vi "Export Waveforms To Spreadsheet File with modified timestamps.vi"(0 "file path (dialog if empty)":path, 1 "prompt":string="Choose file to write.", 3 "delimiter (Tab)":string="\t", 5 "waveforms":waveform(dbl)[](array[waveform]), 7 "error in (no error)":errorcluster, 9 "multiple time columns? (single:F)":bool, 11 "trial start time":timestamp, 12 "append to file? (new file:F)":bool, 14 "header? (write header:T)":bool=TRUE) -> (4 "new file path (Not A Path if cancelled)":path, 15 "error out":errorcluster)   [LabVIEW 2016]
doc: "Converts a waveform to a text string and writes the string to a new byte stream file or appends the string to an existing file. Wire data to the <B>waveforms</B> input to determine the polymorphic instance to use or manually select the instance."
uses:
  <vilib>/Waveform/WDTOps.llb/WDT Get Waveform Time Array DBL.vi
panel:
  out "Array":string[](array[string])
  out "spreadsheet string":string
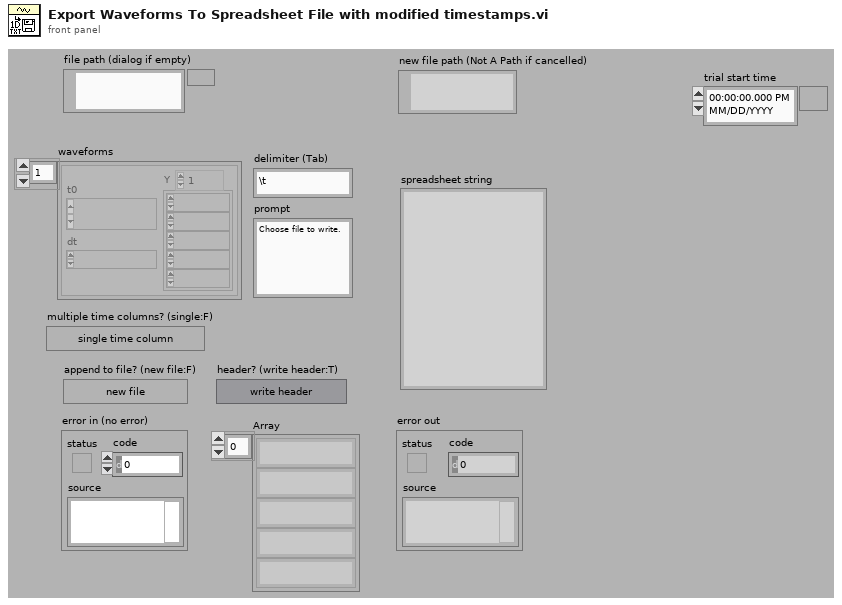
[diagram p1: front panel]
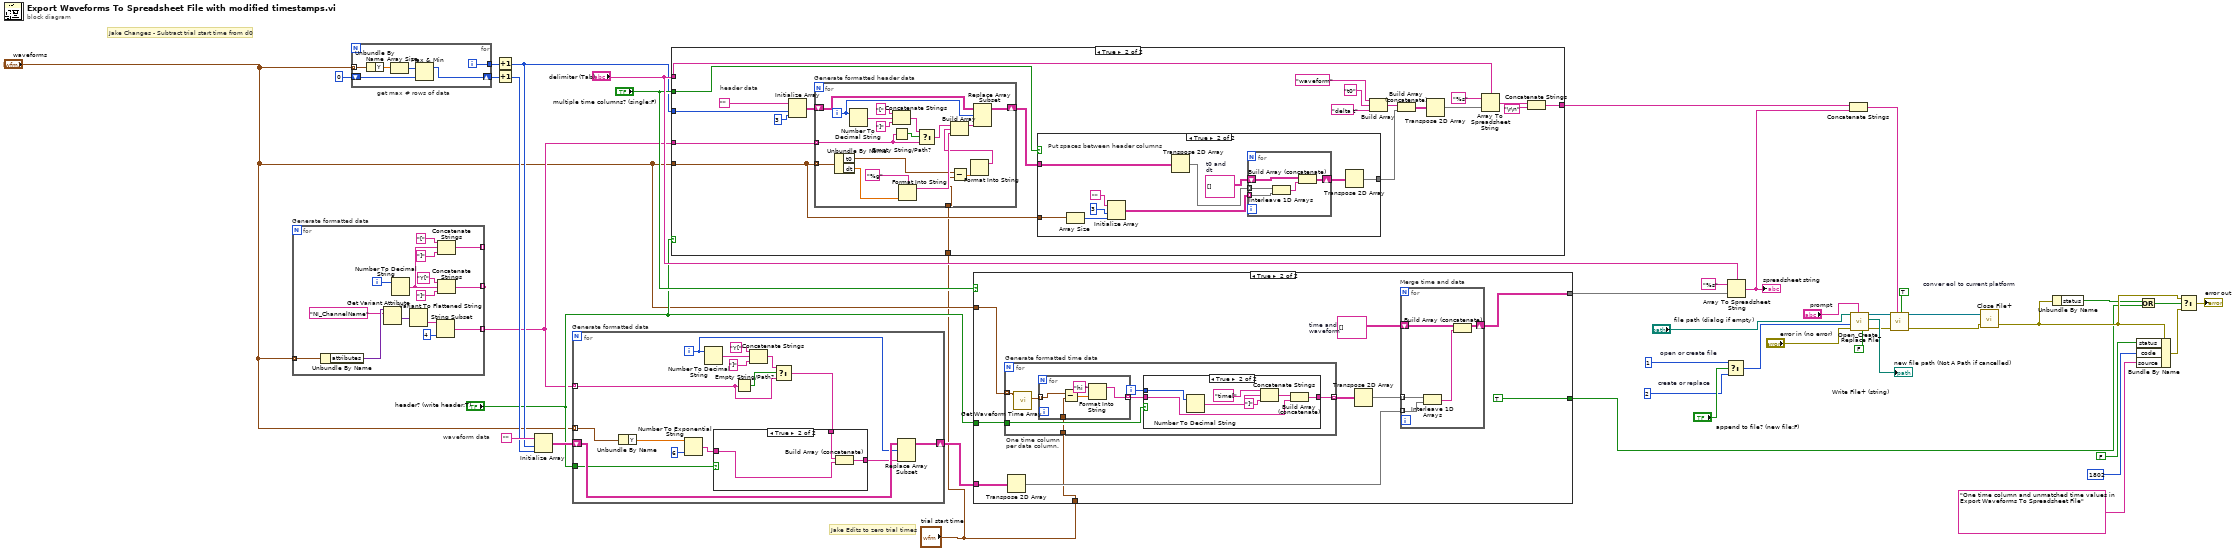
[diagram p0: block diagram]
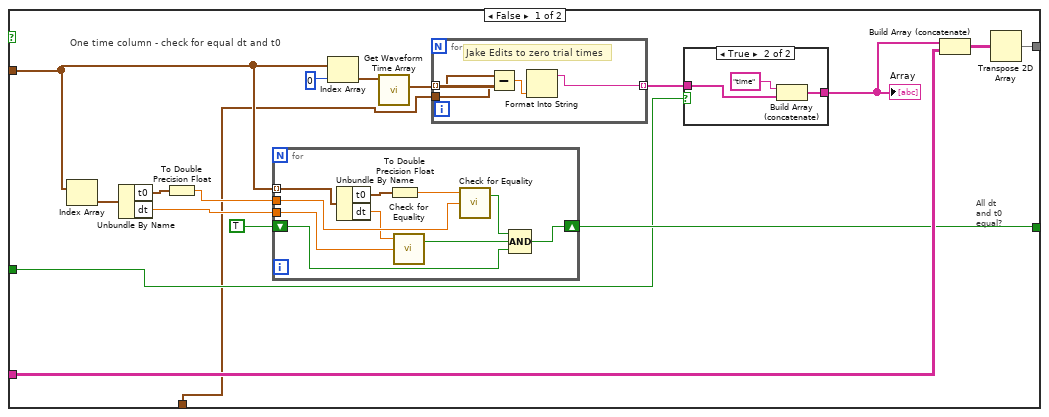
[diagram p2: hidden frame]
diagram:
  w34 = i16 2  # create or replace
  w36 = TRUE  # conver eol to current platform
  w41 = i16 1  # open or create file
  # "Jake Edits to zero trial times"
  # "Jake Changes - Subtract trial start time from d0"
  # "waveform data"
  # "get max # rows of data"
  n1 = for "Generate formatted data" {
    tunnel: "waveforms" -> [w57] mode=indexing
    tunnel: [w48] -> _ mode=indexing
    tunnel: [w47] -> w5 mode=indexing
    tunnel: [w43] -> _ mode=indexing
    i -> [w49]
    n2 = Unbundle By Name(w57) -> ("attributes"=w54:variant)
    n3 = Get Variant Attribute(Variant=w54, name="NI_ChannelName") -> (value=w52:variant)  [unwired: 2 in, 3 out]
    n4 = Number To Decimal String(number=w49) -> (decimal integer string=w44:string)  [unwired: 1 in]
    n5 = Variant To Flattened String(Variant=w52) -> (data string=w55:string)  [unwired: 1 out]
    n6 = String Subset(string=w55, offset (0)=4) -> (substring=w47:string)  [unwired: 1 in]
    n7 = Concatenate Strings("[", w44, "]") -> (w43:string)
    n8 = Concatenate Strings("Y[", w44, "]") -> (w48:string)
  }
  n9 = for {
    tunnel: "waveforms" -> [w63] mode=indexing
    shift-right: [w59] -> w11
    shift-left: 0 -> [w60]
    tunnel: [w58] -> w9
    i -> [w58]
    n10 = Unbundle By Name(w63) -> ("Y"=w62:dbl[])
    n11 = Array Size(array=w62) -> (size(s)=w61:i32)
    n12 = Max & Min(x=w61, y=w60) -> (max(x,y)=w59:i32)  [unwired: 1 out]
  }
  n13 = Increment(x=w9) -> (x+1=w8:i32)
  n14 = Increment(x=w11) -> (x+1=w7:i32)
  n15 = Initialize Array("", w8, w7) -> (w10:string[][])
  n16 = for "Generate formatted data" {
    tunnel: "waveforms" -> [w77] mode=indexing
    tunnel: "header? (write header:T)" -> [w74]
    shift-right: [w75] -> w25
    shift-left: w10 -> [w76]
    tunnel: w5 -> [w64] mode=indexing
    i -> [w66]
    n17 = Unbundle By Name(w77) -> ("Y"=w79:dbl[])
    n18 = Number To Exponential String(number=w79, precision (6)=i16 6) -> (E-format string=w73:string[])  [unwired: 2 in]
    n19 = Number To Decimal String(number=w66) -> (decimal integer string=w71:string)  [unwired: 1 in]
    n20 = Empty String/Path?(string/path=w64) -> (empty?=w68:bool)
    n21 = Concatenate Strings("Y[", w71, "]") -> (w65:string)
    n22 = Select(t=w65, s=w68, f=w64) -> (s? t:f=w67:string)
    n23 = case shown="True" w74 {
      tunnel: w73 -> [w80 w83]
      tunnel: [w80 w82] -> w72
      tunnel: w67 -> [_ w81]
      frame False {
      }
      frame True {
        n24 = Build Array (concatenate)(w81, w83) -> (w82:string[])
      }
    }
    n25 = Replace Array Subset(array=w76, new element=w72, index (row)=w66) -> (w75:string[][])  [unwired: 1 in]
  }
  n26 = case shown="True" "header? (write header:T)" {
    tunnel: "delimiter (Tab)" -> [_ w102]
    tunnel: "waveforms" -> [_ w96]
    tunnel: [_ w97] -> w26
    tunnel: "multiple time columns? (single:F)" -> [_ w94]
    tunnel: w8 -> [_ w87]
    tunnel: w5 -> [_ w85]
    tunnel: "trial start time" -> [_ w84]
    frame False {
    }
    frame True {
      # "header data"
      n27 = Initialize Array("", w87, 3 ("dimension size")) -> (w86:string[][])
      n28 = for "Generate formatted header data" {
        tunnel: w96 -> [w134] mode=indexing
        shift-right: [w130] -> w92
        shift-left: w86 -> [w131]
        tunnel: w85 -> [w125] mode=indexing
        tunnel: w84 -> [w123]
        i -> [w129]
        n29 = Unbundle By Name(w134) -> ("t0"=w122:timestamp, "dt"=w138:dbl)
        n30 = Number To Decimal String(number=w129) -> (decimal integer string=w137:string)  [unwired: 1 in]
        n31 = Concatenate Strings("[", w137, "]") -> (w128:string)
        n32 = Empty String/Path?(string/path=w125) -> (empty?=w126:bool)
        n33 = Format Into String(format string="%g" ("Format String"), w138) -> (resulting string=w139:string)  [unwired: 2 in, 1 out]
        n34 = Select(t=w128, s=w126, f=w125) -> (s? t:f=w127:string)
        n35 = Subtract(x=w122, y=w123) -> (x-y=w124:dbl)
        n36 = Format Into String(w124) -> (resulting string=w121:string)  [unwired: 3 in, 1 out]
        n37 = Build Array(w127, w121, w139) -> (w132:string[])
        n38 = Replace Array Subset(array=w131, new element=w132, index (row)=w129) -> (w130:string[][])  [unwired: 1 in]
      }
      n39 = case shown="True" w94 {
        tunnel: w96 -> [_ w115]
        tunnel: [w105 w110] -> w93
        tunnel: w92 -> [w105 w109]
        frame False {
          # "Leave the header data alone"
        }
        frame True {
          w113 = string[][] []  # t0 and dt
          # "Put spaces between header columns"
          n40 = Array Size(array=w115) -> (size(s)=w106:i32)
          n41 = Initialize Array("", 3 ("Dimension Size"), w106) -> (w112:string[][])
          n42 = Transpose 2D Array(2D array=w109) -> (transposed array=w108:string[][])
          n43 = for {
            shift-right: [w117] -> w111
            shift-left: w113 -> [w118]
            tunnel: w112 -> [w120] mode=indexing
            tunnel: w108 -> [w116] mode=indexing
            n44 = Interleave 1D Arrays(w116, w120) -> (w119:string[])
            n45 = Build Array (concatenate)(w118, w119) -> (w117:string[][])
          }
          n46 = Transpose 2D Array(2D array=w111) -> (transposed array=w110:string[][])
        }
      }
      n47 = Build Array("waveform", "t0", "delta t") -> (w95:string[])
      n48 = Build Array (concatenate)(w95, w93) -> (w90:string[][])
      n49 = Transpose 2D Array(2D array=w90) -> (transposed array=w91:string[][])
      n50 = Array To Spreadsheet String(delimiter (Tab)=w102, array=w91, 3:"%s" ("format string")) -> (spreadsheet string=w99:string)
      n51 = Concatenate Strings(w99, "\r\n") -> (w97:string)
    }
  }
  n52 = case shown="True" "multiple time columns? (single:F)" {
    tunnel: "waveforms" -> [w145 w184]
    tunnel: w25 -> [w152 w182]
    tunnel: [w150 w178] -> w24
    tunnel: [w144 TRUE] -> w14
    tunnel: "header? (write header:T)" -> [w141 w176]
    tunnel: "trial start time" -> [w140 w175]
    frame False {
      # "One time column - check for equal dt and t0"
      # "All dt\nand t0\nequal?"
      n53 = Index Array(array=w145) -> (element=w149:waveform(dbl))  [unwired: 1 in]
      n54 = Unbundle By Name(w149) -> ("t0"=w143:timestamp, "dt"=w146:dbl)
      n55 = To Double Precision Float(number=w143) -> (double precision float=w147:dbl)
      n56 = for {
        tunnel: w145 -> [w170] mode=indexing
        shift-right: [w165] -> w144
        shift-left: TRUE -> [w164]
        tunnel: w147 -> [w168]
        tunnel: w146 -> [w166]
        n57 = Unbundle By Name(w170) -> ("t0"=w161:timestamp, "dt"=w167:dbl)
        n58 = To Double Precision Float(number=w161) -> (double precision float=w169:dbl)
        n59 = call <vilib>:"Check for Equality.vi"("n2"=w166, "n1"=w167) -> ("equal?"=w163:bool)  [unwired: 1 in, 1 out]
        n60 = call <vilib>:"Check for Equality.vi"("n2"=w168, "n1"=w169) -> ("equal?"=w162:bool)  [unwired: 1 in, 1 out]
        n61 = Compound Arithmetic op=AND(w162, w163, w164) -> (w165:bool)
      }
      n62 = Index Array(array=w145, index=0 ("Index")) -> (element=w154:waveform(dbl))
      n63 = call-poly <vilib>:"Get Waveform Time Array.vi"("waveform in"=w154) -> ("X array"=w156:timestamp[])  [unwired: 9 in, 1 out]
      n64 = for {
        tunnel: w156 -> [w173] mode=indexing
        tunnel: [w171] -> w153 mode=indexing
        tunnel: w140 -> [w174]
        # "Jake Edits to zero trial times"
        n65 = Subtract(x=w173, y=w174) -> (x-y=w172:dbl)
        n66 = Format Into String(w172) -> (resulting string=w171:string)  [unwired: 3 in, 1 out]
      }
      n67 = case shown="True" w141 {
        tunnel: w153 -> [w157 w160]
        tunnel: [w157 w159] -> w142
        frame False {
        }
        frame True {
          n68 = Build Array (concatenate)("time", w160) -> (w159:string[])
        }
      }
      "Array" <- w142
      n69 = Build Array (concatenate)(w142, w152) -> (w151:string[][])
      n70 = Transpose 2D Array(2D array=w151) -> (transposed array=w150:string[][])
    }
    frame True {
      w179 = string[][] []  # time and waveform
      # "One time column\nper data column."
      n71 = for "Generate formatted time data" {
        tunnel: [w191] -> w183 mode=indexing
        tunnel: w184 -> [w195] mode=indexing
        tunnel: w176 -> [w193]
        tunnel: w175 -> [w190]
        i -> [w194]
        n72 = call-poly <vilib>:"Get Waveform Time Array.vi"("waveform in"=w195) -> ("X array"=w196:timestamp[])  [unwired: 9 in, 1 out]
        n73 = for {
          tunnel: w196 -> [w208] mode=indexing
          tunnel: [w206] -> w192 mode=indexing
          tunnel: w190 -> [w209]
          n74 = Subtract(x=w208, y=w209) -> (x-y=w207:dbl)
          n75 = Format Into String(initial string="hi ", w207) -> (resulting string=w206:string)  [unwired: 2 in, 1 out]
        }
        n76 = case shown="True" w193 {
          tunnel: w194 -> [_ w201]
          tunnel: w192 -> [w197 w199]
          tunnel: [w197 w198] -> w191
          frame False {
          }
          frame True {
            n77 = Number To Decimal String(number=w201) -> (decimal integer string=w204:string)  [unwired: 1 in]
            n78 = Concatenate Strings("time[", w204, "]") -> (w200:string)
            n79 = Build Array (concatenate)(w200, w199) -> (w198:string[])
          }
        }
      }
      n80 = Transpose 2D Array(2D array=w182) -> (transposed array=w181:string[][])
      n81 = Transpose 2D Array(2D array=w183) -> (transposed array=w180:string[][])
      n82 = for "Merge time and data" {
        tunnel: w181 -> [w188] mode=indexing
        tunnel: w180 -> [w187] mode=indexing
        shift-right: [w186] -> w178
        shift-left: w179 -> [w189]
        n83 = Interleave 1D Arrays(w187, w188) -> (w185:string[])
        n84 = Build Array (concatenate)(w189, w185) -> (w186:string[][])
      }
    }
  }
  n85 = Select ("function")(t=w41, s="append to file? (new file:F)", f=w34) -> (s? t:f=w39:i16)
  n86 = Array To Spreadsheet String(delimiter (Tab)="delimiter (Tab)", array=w24, 3:"%s" ("format (%.3f)")) -> (spreadsheet string=w27:string)
  "spreadsheet string" <- w27
  n87 = Concatenate Strings(w26, w27) -> (w3:string)
  n88 = call <vilib>:"Open_Create_Replace File.vi"("advisory dialog? (display:T)"=FALSE, "prompt"="prompt", "error in (no error)"="error in (no error)", "function (open:0)"=w39, "file path"="file path (dialog if empty)") -> ("error out"=w29:errorcluster, "new file path"=→"new file path (Not A Path if cancelled)":path, "refnum"=w28:refnum<file>)  [unwired: 3 in, 1 out]
  n89 = call <vilib>:"Write File+ (string).vi"("convert eol? (no:F)"=w36, "string"=w3, "error in (no error)"=w29, "refnum"=w28) -> ("error out"=w40:errorcluster, "dup refnum"=w37:refnum<file>)  [unwired: 3 in, 1 out]
  n90 = call <vilib>:"Close File+.vi"("error in (no error)"=w40, "refnum"=w37) -> ("error out"=w21:errorcluster)  [unwired: 3 in, 2 out]
  n91 = Unbundle By Name(w21) -> ("status"=w20:bool)
  n92 = Bundle By Name(cluster=w21, "status"=FALSE, "code"=1802, "source"="One time column and unmatched time values in Export Waveforms To Spreadsheet File") -> (w22:errorcluster)
  n93 = Or(x=w20, y=w14) -> (x .or. y?=w19:bool)
  n94 = Select(t=w21, s=w19, f=w22) -> (s? t:f=→"error out":errorcluster)
